vi "Revision Query.vi"(0 "VISA resource name":refnum<visa-resource-name>, 11 "error in (no error)":errorcluster) -> (4 "VISA resource name out":refnum<visa-resource-name>, 8 "Instr Driver Revision":string, 10 "Instr Firmware Revision":string, 15 "error out":errorcluster)   [LabVIEW 2011, in "Fluke 5XXX Series Multicalibrators.lvlib"]
doc: "This VI queries the current instrument firmware revision and instrument driver revision.\n\nThis Instrument Driver's Revision number is Rev 1.0, 09/2002, LV 5.1 and is tested with instrument model 5500A, main firmware version 2.5, encoder firmware 1.3, inguard firmware 2.0, and 5725A not attached.\n\nFluke 5xxx Series Multi-Calibrator instrument driver\nCreated By: Petr Marcalik, ELCOM a.s., DVI, Czech Republic\nRelease Date: September 2002\nOriginally Developed in LabVIEW Version: 5.1\n\nModification History: \n\nNone"
uses:
  Fluke 5XXX Series Multicalibrators.lvlib
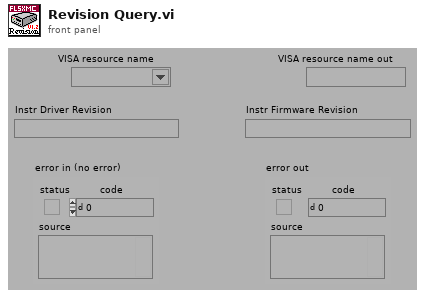
[diagram p1: front panel]
types:
  T1 = enum32{"invalid app kind", "Development System", "Run Time System", "Student Edition", "Embedded LabVIEW", "Evaluation", "Custom"}
  T2 = cluster{"Major":u16, "Minor":u16, "Fix":u16, "Build":u16}
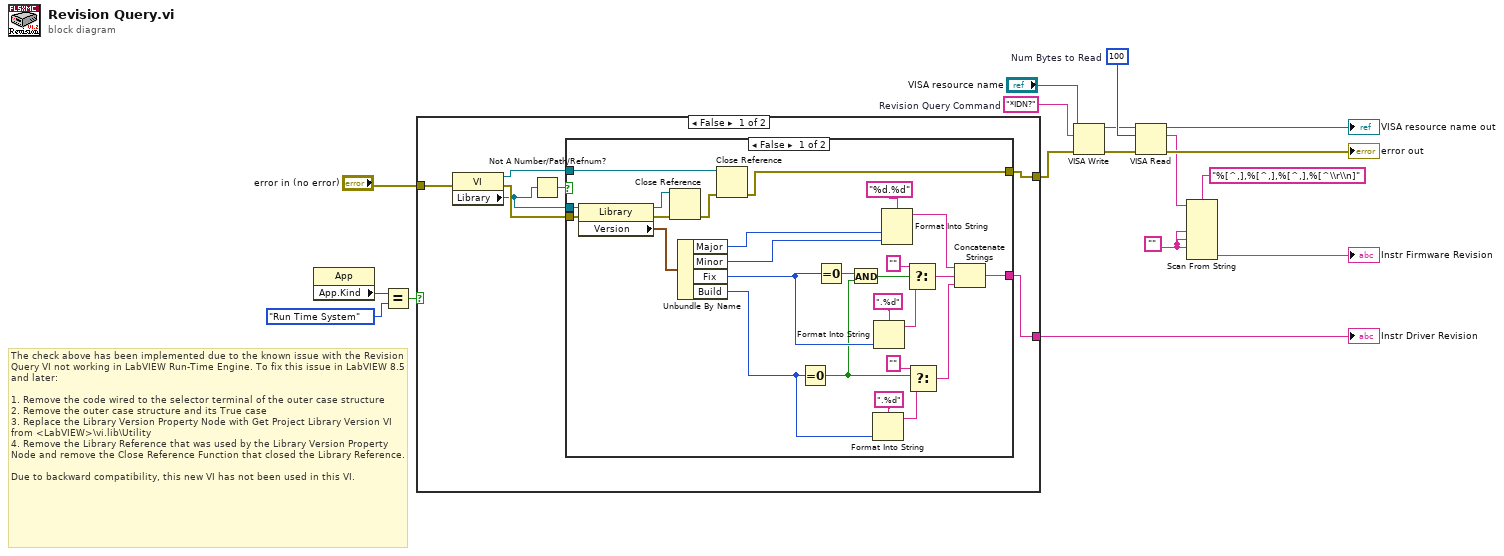
[diagram p0: block diagram]
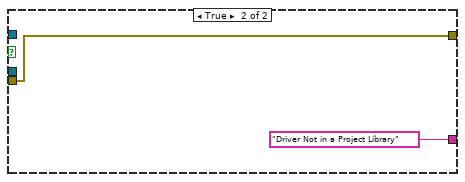
[diagram p2: hidden frame]
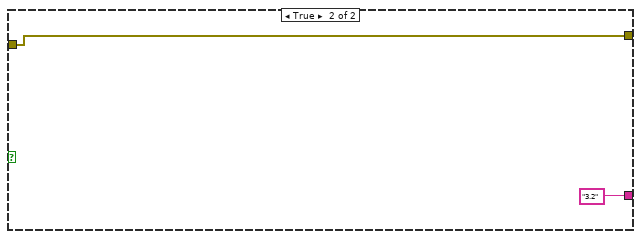
[diagram p3: hidden frame]
diagram:
  w8 = ""
  w11 = "*IDN?"  # Revision Query Command
  w14 = u32 100  # Num Bytes to Read
  # "The check above has been implemented due to the known issue with the Revision Query VI not working in LabVIEW Run-Time Engine. To fix this issue in LabVIEW 8.5 and later:\n\n1. Remove the code wired to the selector terminal of the outer case structure\n2. Remove the outer case structure and its True case\n3. Replace the Library Version Property Node with Get Project Library Version VI from <LabVIEW>\\vi.lib\\Utility\n4. Remove the Library Reference that was used by the Library Version Property Node and remove the Close Reference Function that closed the Library Reference.\n\nDue to backward compatibility, this new VI has not been used in this VI."
  n1 = property class="App"() -> ("App.Kind"=w2:T1)  [unwired: 2 in, 2 out]
  n2 = Equal?(x=w2, y=T1."Run Time System") -> (x = y?=w3:bool)
  n3 = case shown="False" w3 {
    tunnel: "error in (no error)" -> [w24 w54]
    tunnel: [w19 "3.2"] -> w5
    tunnel: [w18 w54] -> w4
    frame False {
      n4 = property class="VI"(error in=w24) -> (reference out=w20:refnum<vi>, error out=w23:errorcluster, "Library"=w22:refnum<vi>)  [unwired: 1 in]
      n5 = Not A Number/Path/Refnum?(number/path/refnum=w22) -> (NaN/Path/Refnum?=w21:bool)
      n6 = case shown="False" w21 {
        tunnel: [w29 w51] -> w18
        tunnel: [w28 "Driver Not in a Project Library"] -> w19
        tunnel: w23 -> [w27 w51]
        tunnel: w22 -> [w26 _]
        tunnel: w20 -> [w25 _]
        frame False {
          n7 = property class="Library"(reference=w26, error in=w27) -> (reference out=w49:refnum<vi>, error out=w50:errorcluster, "Version"=w47:T2)
          n8 = Close Reference(reference=w49, error in (no error)=w50) -> (error out=w48:errorcluster)
          n9 = Unbundle By Name(w47) -> ("Major"=w36:u16, "Minor"=w35:u16, "Fix"=w33:u16, "Build"=w34:u16)
          n10 = Close Reference(reference=w25, error in (no error)=w48) -> (error out=w29:errorcluster)
          n11 = Equal To 0?(x=w34) -> (x = 0?=w31:bool)
          n12 = Equal To 0?(x=w33) -> (x = 0?=w32:bool)
          n13 = And(x=w32, y=w31) -> (x .and. y?=w30:bool)
          n14 = Format Into String(format string=".%d", w34) -> (resulting string=w40:string)  [unwired: 2 in, 1 out]
          n15 = Format Into String(format string=".%d", w33) -> (resulting string=w44:string)  [unwired: 2 in, 1 out]
          n16 = Format Into String(format string="%d.%d", w36, w35) -> (resulting string=w42:string)  [unwired: 2 in, 1 out]
          n17 = Select(t="", s=w30, f=w44) -> (s? t:f=w41:string)
          n18 = Select(t="", s=w31, f=w40) -> (s? t:f=w37:string)
          n19 = Concatenate Strings(w42, w41, w37) -> (w28:string)
        }
        frame True {
        }
      }
    }
    frame True {
    }
  }
  "Instr Driver Revision" <- w5
  n20 = VISA Write(VISA resource name="VISA resource name", write buffer=w11, error in (no error)=w4) -> (VISA resource name out=w13:refnum<visa-resource-name>, error out=w12:errorcluster)  [unwired: 1 out]
  n21 = VISA Read(VISA resource name=w13, byte count=w14, error in (no error)=w12) -> (VISA resource name out=→"VISA resource name out":refnum<visa-resource-name>, read buffer=w10:string, error out=→"error out":errorcluster)  [unwired: 1 out]
  n22 = Scan From String(format string="%[^,],%[^,],%[^,],%[^\\r\\n]", input string=w10, default 1=w8, default 2=w8, default 3=w8) -> (output 4=→"Instr Firmware Revision":string)  [unwired: 6 in, 3 out]
